vi "ex04 - размер пакета данных.vi"() -> ()   [LabVIEW 2009]
uses:
  Z210/Z210 CTL Lib.llb/Z210 CTL ADC Inputs Status.ctl
  Z210/Z210 CTL Lib.llb/Z210 CTL ADC Channel Type.ctl
  Z210/Z210 CTL Lib.llb/Z210 CTL DAC Inputs Status.ctl
  Z210/Z210 CTL Lib.llb/Z210 CTL ADC or DAC Function.ctl
panel:
  out "размер пакета данных\nby Z210 DATA AD Get Packet Size":i32
  in  "AorD":T1
  out "Inputs Status DAC":T2
  out "частота дискр. АЦП/ЦАП\nby R SetFrequency":dbl[unit]
  out "размер буфера данных\nby ROUTINE Allocate Buffer":i32 format="%x"
  out "bufferAddr\nby ROUTINE Allocate Buffer":u32 format="%x"
  out "Inputs Status ADC":T3
  in  "N ЦАП (0)":i32
  in  "N Синф (0)":i32
  in  "N Дифф (0)":i32
  in  "stop":bool
  out "Размеры пакетов (words)\nby Get Pointer":i32[](array[numeric])
  out "максимальный размер внутреннего буффера устройства\nby Z210 DATA AD Get DeviceBuffer Max Size":i32
  # "размер пакета данных \nи\nразмер внутреннего буффера устройства"
  # "СПРАВОЧНО:"
  # "1. Выбрать АЦП/ЦАП.\n2. Включить каналы (ниже). Не важно какие именно,\nглавное чтобы хотя бы один был включен.\n3. Смотреть размеры.\n4. Нажать стоп."
  # "Включить каналы:"
  # "В моем случае размер внутреннего буффера устройства\nсовпадает с размером пакета.\n\nАЦП 4032 words (max 16128)\nЦАП 4096 words (max 16384)\n\nВсе размеры даны в 16-битных словах"
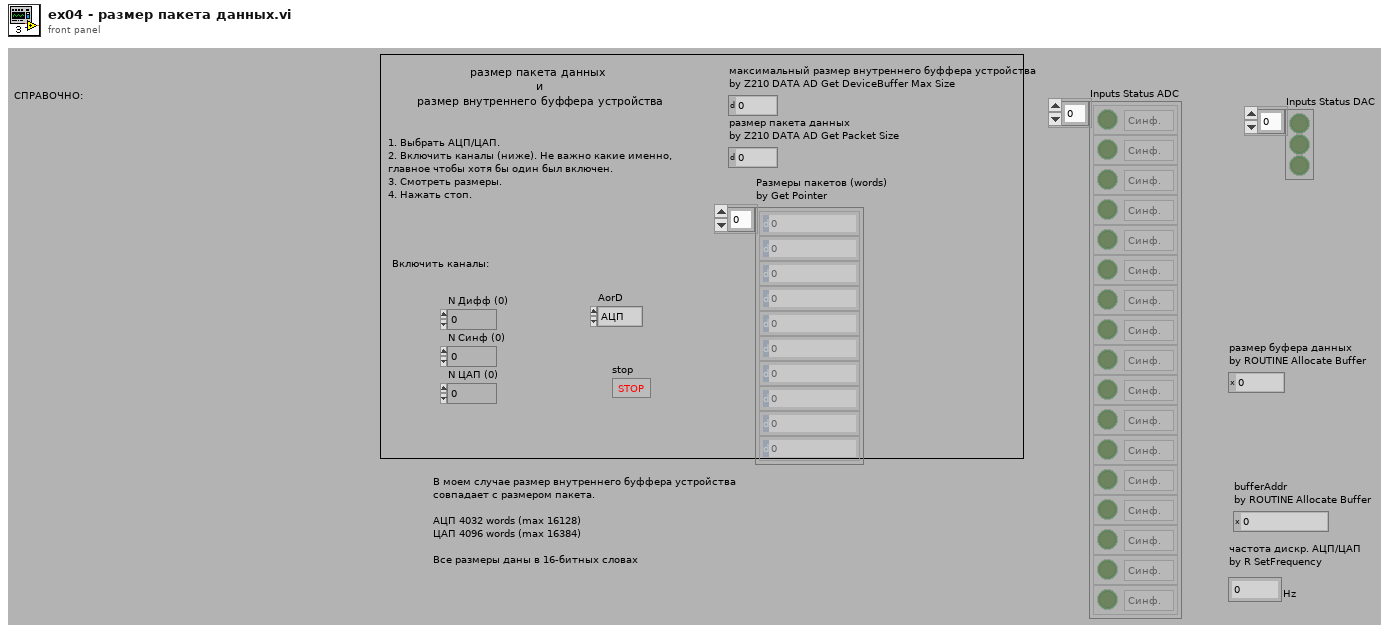
[diagram p1: front panel]
types:
  T1 = typedef "Z210 CTL ADC or DAC Function.ctl" = enum16{"АЦП", "ЦАП", "Both"}
  T2 = typedef "Z210 CTL DAC Inputs Status.ctl" = bool[]
  T3 = typedef "Z210 CTL ADC Inputs Status.ctl" = cluster{"isEnabled?":bool, "ADCchType":T4}[]
  T4 = typedef "Z210 CTL ADC Channel Type.ctl" = enum16{"Синф.", "Дифф."}
  T5 = typedef "Z210 CTL Unit Data .ctl" = cluster{"typeDevice":i32, "numberDSP":i32}
  T6 = typedef "Z210 CTL Buffers Params.ctl" = cluster{"bufferAddr ADC":u32, "bufferSize ADC":i32, "bufferAddr DAC":u32, "bufferSize DAC":i32}
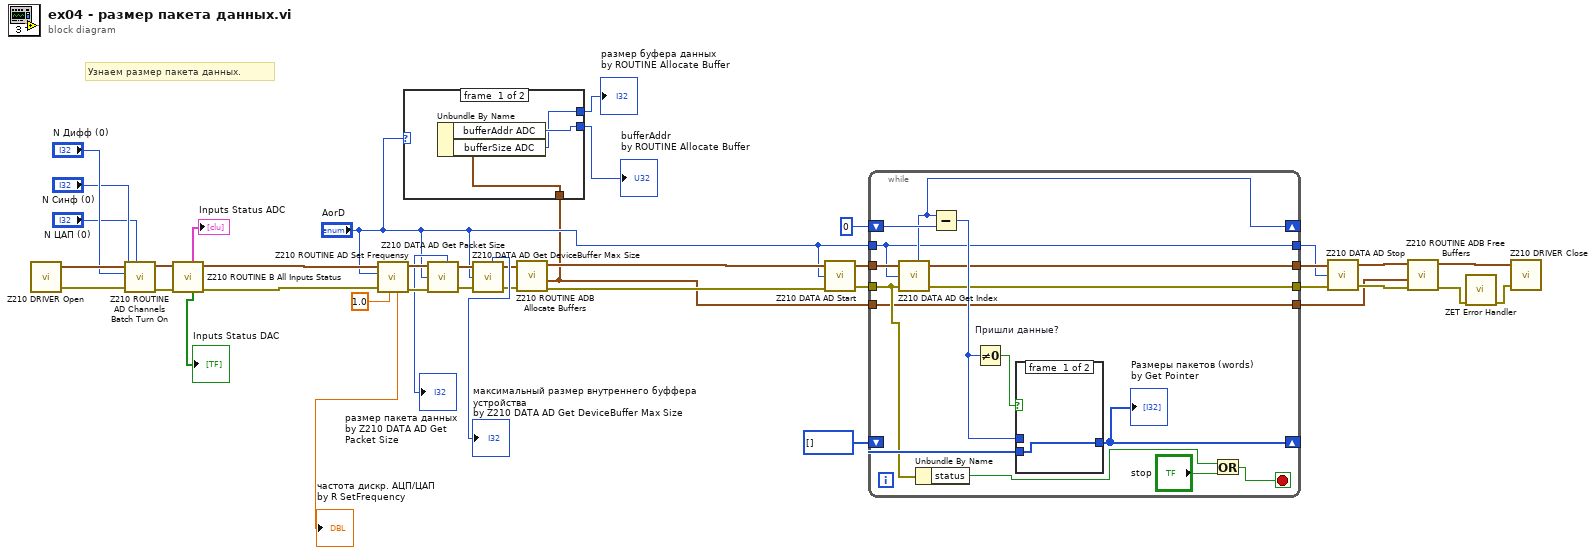
[diagram p0: block diagram]
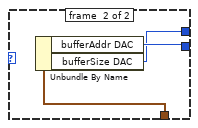
[diagram p2: hidden frame]
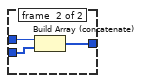
[diagram p3: hidden frame]
diagram:
  # "Узнаем размер пакета данных."
  n1 = call "Z210 DRIVER Open.vi"() -> ("unitData out"=w40:T5, "error IO"=w39:errorcluster)  [unwired: 8 in]
  n2 = call "Z210 ROUTINE AD Channels Batch Turn On.vi"("N ЦАП (0)"="N ЦАП (0)", "error in (no error)"=w39, "N Синф (0)"="N Синф (0)", "N Дифф (0)"="N Дифф (0)", "unitData in"=w40) -> ("error out"=w37:errorcluster, "unitData out"=w38:T5)  [unwired: 3 in, 2 out]
  n3 = call "Z210 ROUTINE B All Inputs Status.vi"("error in (no error)"=w37, "unitData in"=w38) -> ("error out"=w10:errorcluster, "unitData out"=w11:T5, "Inputs Status DAC"=→"Inputs Status DAC":T2, "Inputs Status ADC"=→"Inputs Status ADC":T3)  [unwired: 6 in]
  n4 = call "Z210 ROUTINE AD Set Frequensy.vi"("freq suggestion"=dbl[unit] 1.0, "error in (no error)"=w10, "AorD"="AorD", "unitData in"=w11) -> ("error out"=w16:errorcluster, "unitData out"=w17:T5, "freq"=→"частота дискр. АЦП/ЦАП\nby R SetFrequency":dbl[unit])  [unwired: 5 in]
  n5 = call "Z210 DATA AD Get Packet Size.vi"("unitData in"=w17, "AorD"="AorD", "error in (no error)"=w16) -> ("packetSize"=→"размер пакета данных\nby Z210 DATA AD Get Packet Size":i32, "unitData out"=w15:T5, "error out"=w14:errorcluster)  [unwired: 4 in]
  n6 = call "Z210 DATA AD Get DeviceBuffer Max Size.vi"("unitData in"=w15, "AorD"="AorD", "error in (no error)"=w14) -> ("unitData out"=w9:T5, "size"=→"максимальный размер внутреннего буффера устройства\nby Z210 DATA AD Get DeviceBuffer Max Size":i32, "error out"=w8:errorcluster)  [unwired: 4 in]
  n7 = call "Z210 ROUTINE ADB Allocate Buffers.vi"("error in (no error)"=w8, "unitData in"=w9) -> ("error out"=w6:errorcluster, "buffersParams out"=w2:T6, "unitData out"=w7:T5)  [unwired: 7 in]
  n8 = case shown="\"АЦП\", Default" "AorD" {
    tunnel: w2 -> [w43 w46]
    tunnel: [w42 w45] -> w4
    tunnel: [w41 w44] -> w3
    frame #0 {
      n9 = Unbundle By Name(w43) -> ("bufferAddr ADC"=w42:u32, "bufferSize ADC"=w41:i32)
    }
    frame #1 {
      n10 = Unbundle By Name(w46) -> ("bufferAddr DAC"=w45:u32, "bufferSize DAC"=w44:i32)
    }
  }
  "bufferAddr\nby ROUTINE Allocate Buffer" <- w4
  "размер буфера данных\nby ROUTINE Allocate Buffer" <- w3
  n11 = call "Z210 DATA AD Start.vi"("unitData in"=w7, "AorD"="AorD", "error in (no error)"=w6) -> ("unitData out"=w28:T5, "error out"=w27:errorcluster)  [unwired: 5 in]
  n12 = while {
    tunnel: w28 -> [w61]
    tunnel: "AorD" -> [w54]
    tunnel: w27 -> [w53]
    shift-right: [w59] -> _
    shift-left: 0 ("pointer") -> [w60]
    shift-right: [w56] -> _
    shift-left: i32[] [] -> [w55]
    tunnel: [w49] -> w26
    tunnel: [w48] -> w25
    tunnel: [w54] -> w22
    tunnel: w2 -> [w47]
    tunnel: [w47] -> w1
    stop <- w50 stop-if-true
    n13 = call "Z210 DATA AD Get Index.vi"("unitData in"=w61, "AorD"=w54, "error in (no error)"=w53) -> ("index"=w59:i32, "unitData out"=w49:T5, "error out"=w48:errorcluster)  [unwired: 4 in]
    n14 = Unbundle By Name(w53) -> ("status"=w51:bool)
    n15 = Subtract(x=w59, y=w60) -> (x-y=w57:i32)
    n16 = Not Equal To 0? "Пришли данные?"(x=w57) -> (x != 0?=w58:bool)
    n17 = case shown="False" w58 {
      tunnel: w57 -> [_ w65]
      tunnel: [w62 w64] -> w56
      tunnel: w55 -> [w62 w63]
      frame #0 {
      }
      frame #1 {
        n18 = Build Array (concatenate)(w65, w63) -> (w64:i32[])
      }
    }
    "Размеры пакетов (words)\nby Get Pointer" <- w56
    n19 = Or(x=w51, y="stop") -> (x .or. y?=w50:bool)
  }
  n20 = call "Z210 DATA AD Stop.vi"("unitData in"=w26, "AorD"=w22, "error in (no error)"=w25) -> ("unitData out"=w24:T5, "error out"=w23:errorcluster)  [unwired: 5 in]
  n21 = call "Z210 ROUTINE ADB Free Buffers.vi"("error in (no error)"=w23, "buffersParams"=w1, "unitData in"=w24) -> ("error out"=w31:errorcluster, "unitData out"=w30:T5)  [unwired: 6 in, 1 out]
  n22 = call "ZET Error Handler.vi"("error in (no error)"=w31) -> ("error out"=w29:errorcluster)  [unwired: 9 in, 1 out]
  n23 = call "Z210 DRIVER Close.vi"("unitData in"=w30, "error in (no error)"=w29) -> ()  [unwired: 6 in, 2 out]
